vi "Big_LED_control.vi"() -> ()   [LabVIEW 2018]
uses:
  <instrlib>/niDCPower/nidcpower.llb/niDCPower Source Mode.ctl
  D:/#msp/LV/LED_CONTROL_big_LED_ophir_19.12_1/AT lib/AmateurStepperMotor.dll
  AT lib/AmateurStepperMotor.dll
  <instrlib>/niDMM/nidmm.llb/niDMM Function.ctl
  <instrlib>/niDMM/nidmm.llb/niDMM Resolution in Digits.ctl
  <instrlib>/niDCPower/nidcpower.llb/niDCPower Measurement Type.ctl
  <vilib>/Instr/_visa.llb/VISA Configure Serial Port (Instr).vi
  <instrlib>/niDMM/nidmm.llb/niDMM Configure Measurement Digits.vi
panel:
  in  "Tab Control 2":enum32{"Шаговик и офир", "Служебная область"}(tab)
  in  "milliseconds to wait":u32=1000
  in  "Go To":dbl
  out "Ophir 1 Char":dbl(graph)=7.0
  in  "DecelerationTime, s":dbl
  in  "AccelerationTime, s":dbl
  in  "HoldOn":bool
  in  "Ophir 1 units":string(combo)="1000" caption="Units"
  out "Ophir 1 Over Range":bool caption="Over Range"
  out "Ophir 1 Optical Power":dbl=7.0 caption="Power" format="%#_4g"
  out "Ophir 1 MAX":dbl=7.0200000000000005 caption="MAX" format="%#_5g"
  in  "Ophir 1 Clear":bool caption="Clear"
  in  "StepMultiplicationFactor":dbl=1.0
  in  "StepDivisor":i32(ring)=8 items=["D1"=1, "D2"=2, "D4"=4, "D8"=8, "D16"=16, "D32"=32]
  in  "Speed":dbl=1000.0
  in  "Погнали!":bool
  in  "Стоп GoTo":bool
  out "Готово":bool
  out "Position":dbl
  in  "Ophir 1 Info":u16(ring)=1 caption="Info" items=["Device : JUNO; s/n:903793", "Head : PD300R-3W   ; s/n:779628"]
  in  "new pos":dbl
  in  "set pos":bool
  out "Device Response":string="*\n"
  in  "Ophir 1 usb channel":i16 caption="usb channel"
  out "Ophir 1 dup Visa Session":refnum<visa-resource-name>="USB0::0x0BD3::0x0777::NI-VISA-60004::RAW" caption="dup Visa Session"
  in  "Ophir 1 Baud Rate (3:9600)":i16(ring)=3 caption="Baud Rate (3:9600)" items=["300", "1200", "4800", "9600", "19200", "38400"]
  out "Ophir 1 Real Optical Power":dbl=0.007 format="%.6e"
  in  "Ophir 1 GPIB Address (10)":string="10" caption="GPIB Address (10)"
  in  "Ophir 1 Port Number (default 2)":i16=1 caption="Port Number (default 2)" min=0 max=20
  in  "Ophir 1 Select Communication Protocol":u16(ring) caption="Select Communication Protocol" items=["USB", "RS232", "GPIB"]
  out "Ophir 1 error out":errorcluster caption="error out"
  in  "Ophir 1 error in (no error)":errorcluster caption="error in (no error)"
  in  "Ophir 1 Wait":u32=100 caption="Wait"
  out "IsOpen":bool=TRUE
  out "Ophir 1 Initialization":bool=TRUE caption="Initialization"
  in  "Tab Control":T1(tab)
  in  "POWER":bool
  in  "Стоп":bool
  in  "Resource Name":refnum<k15>="PXI1Slot2" caption="Источник питания"
  in  "Амперметр":refnum<k15>="PXI1Slot4" caption="NI DMM 1"
  in  "V_MB, V":dbl=5.0 caption="voltage level" format="%_6p"
  in  "curlim_V_MB, A":dbl=0.3 caption="current limit" format="%_6p"
  out "curmes_V_MB, A":dbl caption="measurement" format="%_6g"
  out "chart_0":dbl(graph)=-0.001986406197333734 caption="Waveform Chart 5"
  in  "voltlim_I_LED, V":dbl=2.0 caption="current limit" min=0.01 format="%_6p"
  in  "I_LED, A":dbl=0.005 caption="voltage level" format="%_6p"
  out "chart_1":dbl(graph) caption="Waveform Chart 5"
  out "voltmes_I_LED, V":dbl caption="measurement" format="%_6g"
  out "Current Char":dbl(graph)=0.0019995495676994324
  in  "Arduino":refnum<visa-resource-name>="COM14"
  in  "Сегменты":bool[](array[boolean])=[FALSE, FALSE, FALSE, FALSE, FALSE, FALSE, FALSE, FALSE, FALSE, FALSE, FALSE, FALSE, FALSE, FALSE, FALSE, FALSE, FALSE, FALSE]
  in  "Вольтметр":refnum<k15>="PXI1Slot5" caption="NI DMM 1"
  out "Voltage Char":dbl(graph)=nan
  in  "Port Name":string="COM7" caption="Порт шаговика"
  in  "wave_lenght":string="600"
  in  "Промер":bool caption="Промер сегмента"
  in  "NI DMM 1 Voltage Range 4":string(combo)="-1" caption="Range"
  in  "NI DMM 1 units 4":string(combo)="1" caption="Units"
  out "Voltage":dbl=nan format="%_6g"
  in  "NI DMM 1 Current Range 3":string(combo)="1" caption="Range"
  in  "NI DMM 1 units 3":string(combo)="1000" caption="Units"
  out "Current":dbl=0.0019995495676994324 format="%_6g"
  out "Разряд":dbl
  out "+/-":bool
  out "Power off":bool=TRUE
  in  "Command":string="Anode"
  in  "Записать":bool
  out "measure output file refnum":refnum<file>
  out "Voltage, V":dbl=nan caption="Measurement" format="%.5f"
  out "Current, A":dbl=1.9995495676994324e-06 caption="Measurement" format="%.5f"
  out "Тип индикатора":string="Anode"
  out "chart_2":dbl(graph)=4.286668577189643e-07
  in  "V_RES, V":dbl caption="voltage level" format="%_6p"
  out "curmes_V_RES, A":dbl caption="measurement" format="%_6g"
  in  "curlim_V_RES, A":dbl=0.1 caption="current limit" min=0.01 format="%_6p"
  in  "measure path":path=path "D:/NI LabVIEW/MultiOpto/MultiOpto_1.2/Logs/SEL"
  out "Enum":enum16{"Exit", "4", "Промер", "2", "1"}(ring)
  out "№ об-ца":dbl=-1.0
  out "Темп-ра":dbl=-1.0
  out "Сегмент":string
  # "Шаговик"
  # "Офир"
  # "Шаговик"
  # "Офир"
  # "position - это значение абсолютное"
  # "j"
  # "c"
  # "d"
  # "e"
  # "g"
  # "h"
  # "a"
  # "b"
  # "f"
  # "k"
  # "L"
  # "m"
  # "n"
  # "p"
  # "dp"
  # "all"
  # "V_MB 5 В\nогрничение 300 м\n\nV_LED 2,1 В\nограничение 200 м"
  # "единицы мА\nrange 1 А"
  # "1. каждый сегмент включаем по отдельности, резистором постраиваем ток до 10 мА\n2. напряжение V_LED при этом не меняется\n3. в такоом положении промеряем сегменты по отдельности\n4. для промера всего индикатора сразу подстраиваем напряжение при неизменном положении резисторов\n5. ток всех индикаторов = ток одного сегмента (10 мА) * число сегментов (15)\n6. добиваемся этого увеличением V_LED"
  # "единицы В\nrange AUTO"
  # "регклировка суммарного тока через индикатор"
  # "24.063\n\n     I          U\n20 мА  1.3 В\n20 мА  1.4 В\n 7 мА   1.15 В"
  # "24.064\n\n     I          U\n10 мА  2 В\n10 мА  2.15 В\n 7 мА   1.9 В"
  # "автоматизировать подбор напряжения по известному максимальному напряжению и току. ОС по току сегмента"
  # "Р1:  +25°C\nР2:  - 60°C\nР3:  +85°C"
  # "регулировать ток в зависимости от температуры.\nс ростом температуры растет ток.\nпид-регулятор??"
  # "0. ввести номер образца\n1. включить нужный сегмент\n2. ввести его в поле справа\n3. вести температуру в поле слева\n4. нажать кнопку \"промер сегмента\""
  # "\"опрашивать кнопки не чаще, чем раз в секунду. сейчас кликать можно чаще, они загорятся, но ничего не произойдет\""
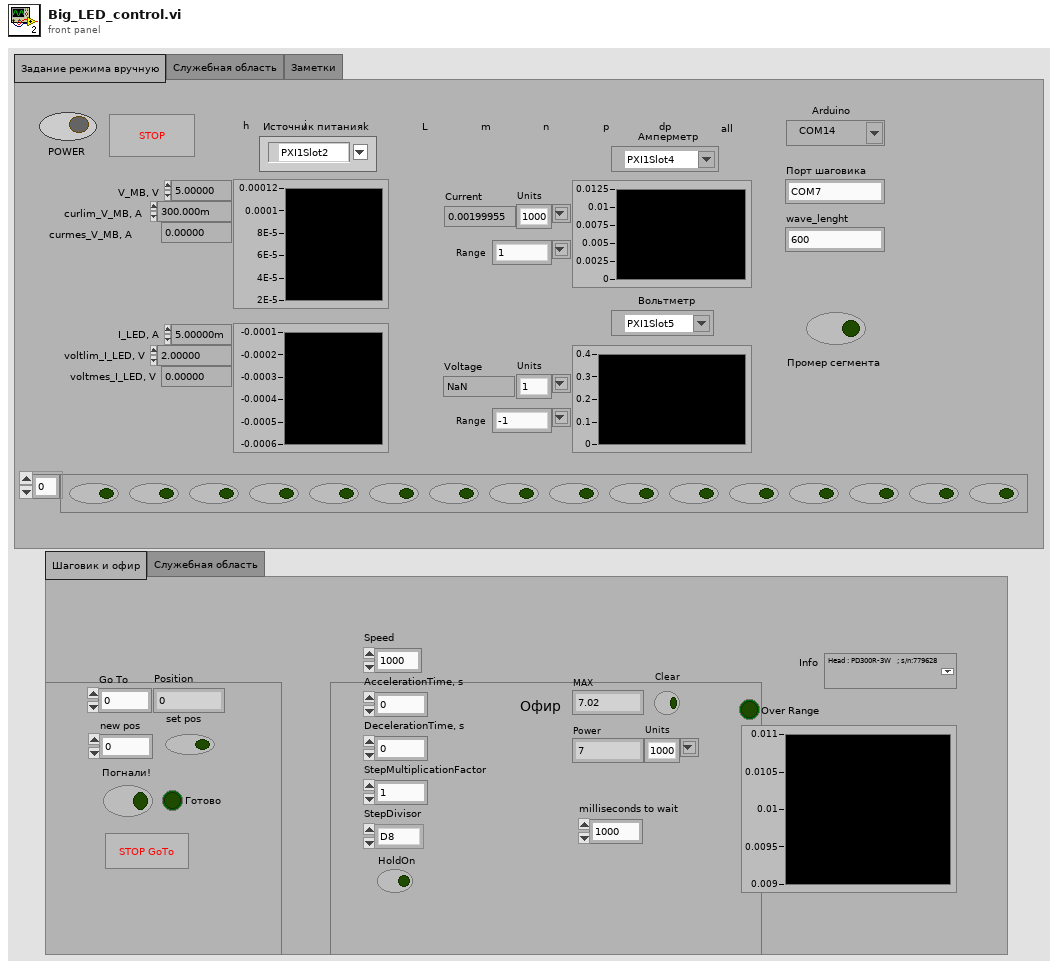
[diagram p1: front panel]
types:
  T1 = enum32{"Задание режима вручную", "Служебная область", "Заметки"}
  T2 = enum16{"open", "replace", "create", "open or create", "replace or create", "replace or create with confirmation"}
  T3 = typedef "niDCPower Source Mode.ctl" = i32
  T4 = typedef "niDCPower Measurement Type.ctl" = i32
  T5 = typedef "niDMM Function.ctl" = enum16{"DC Volts", "AC Volts", "DC Current", "AC Current", "2-wire Resistance", "4-wire Resistance", "Diode", "Frequency", "Period", "AC Volts DC Coupled", "Capacitance", "Inductance", "Temperature"}
  T6 = typedef "niDMM Resolution in Digits.ctl" = dbl
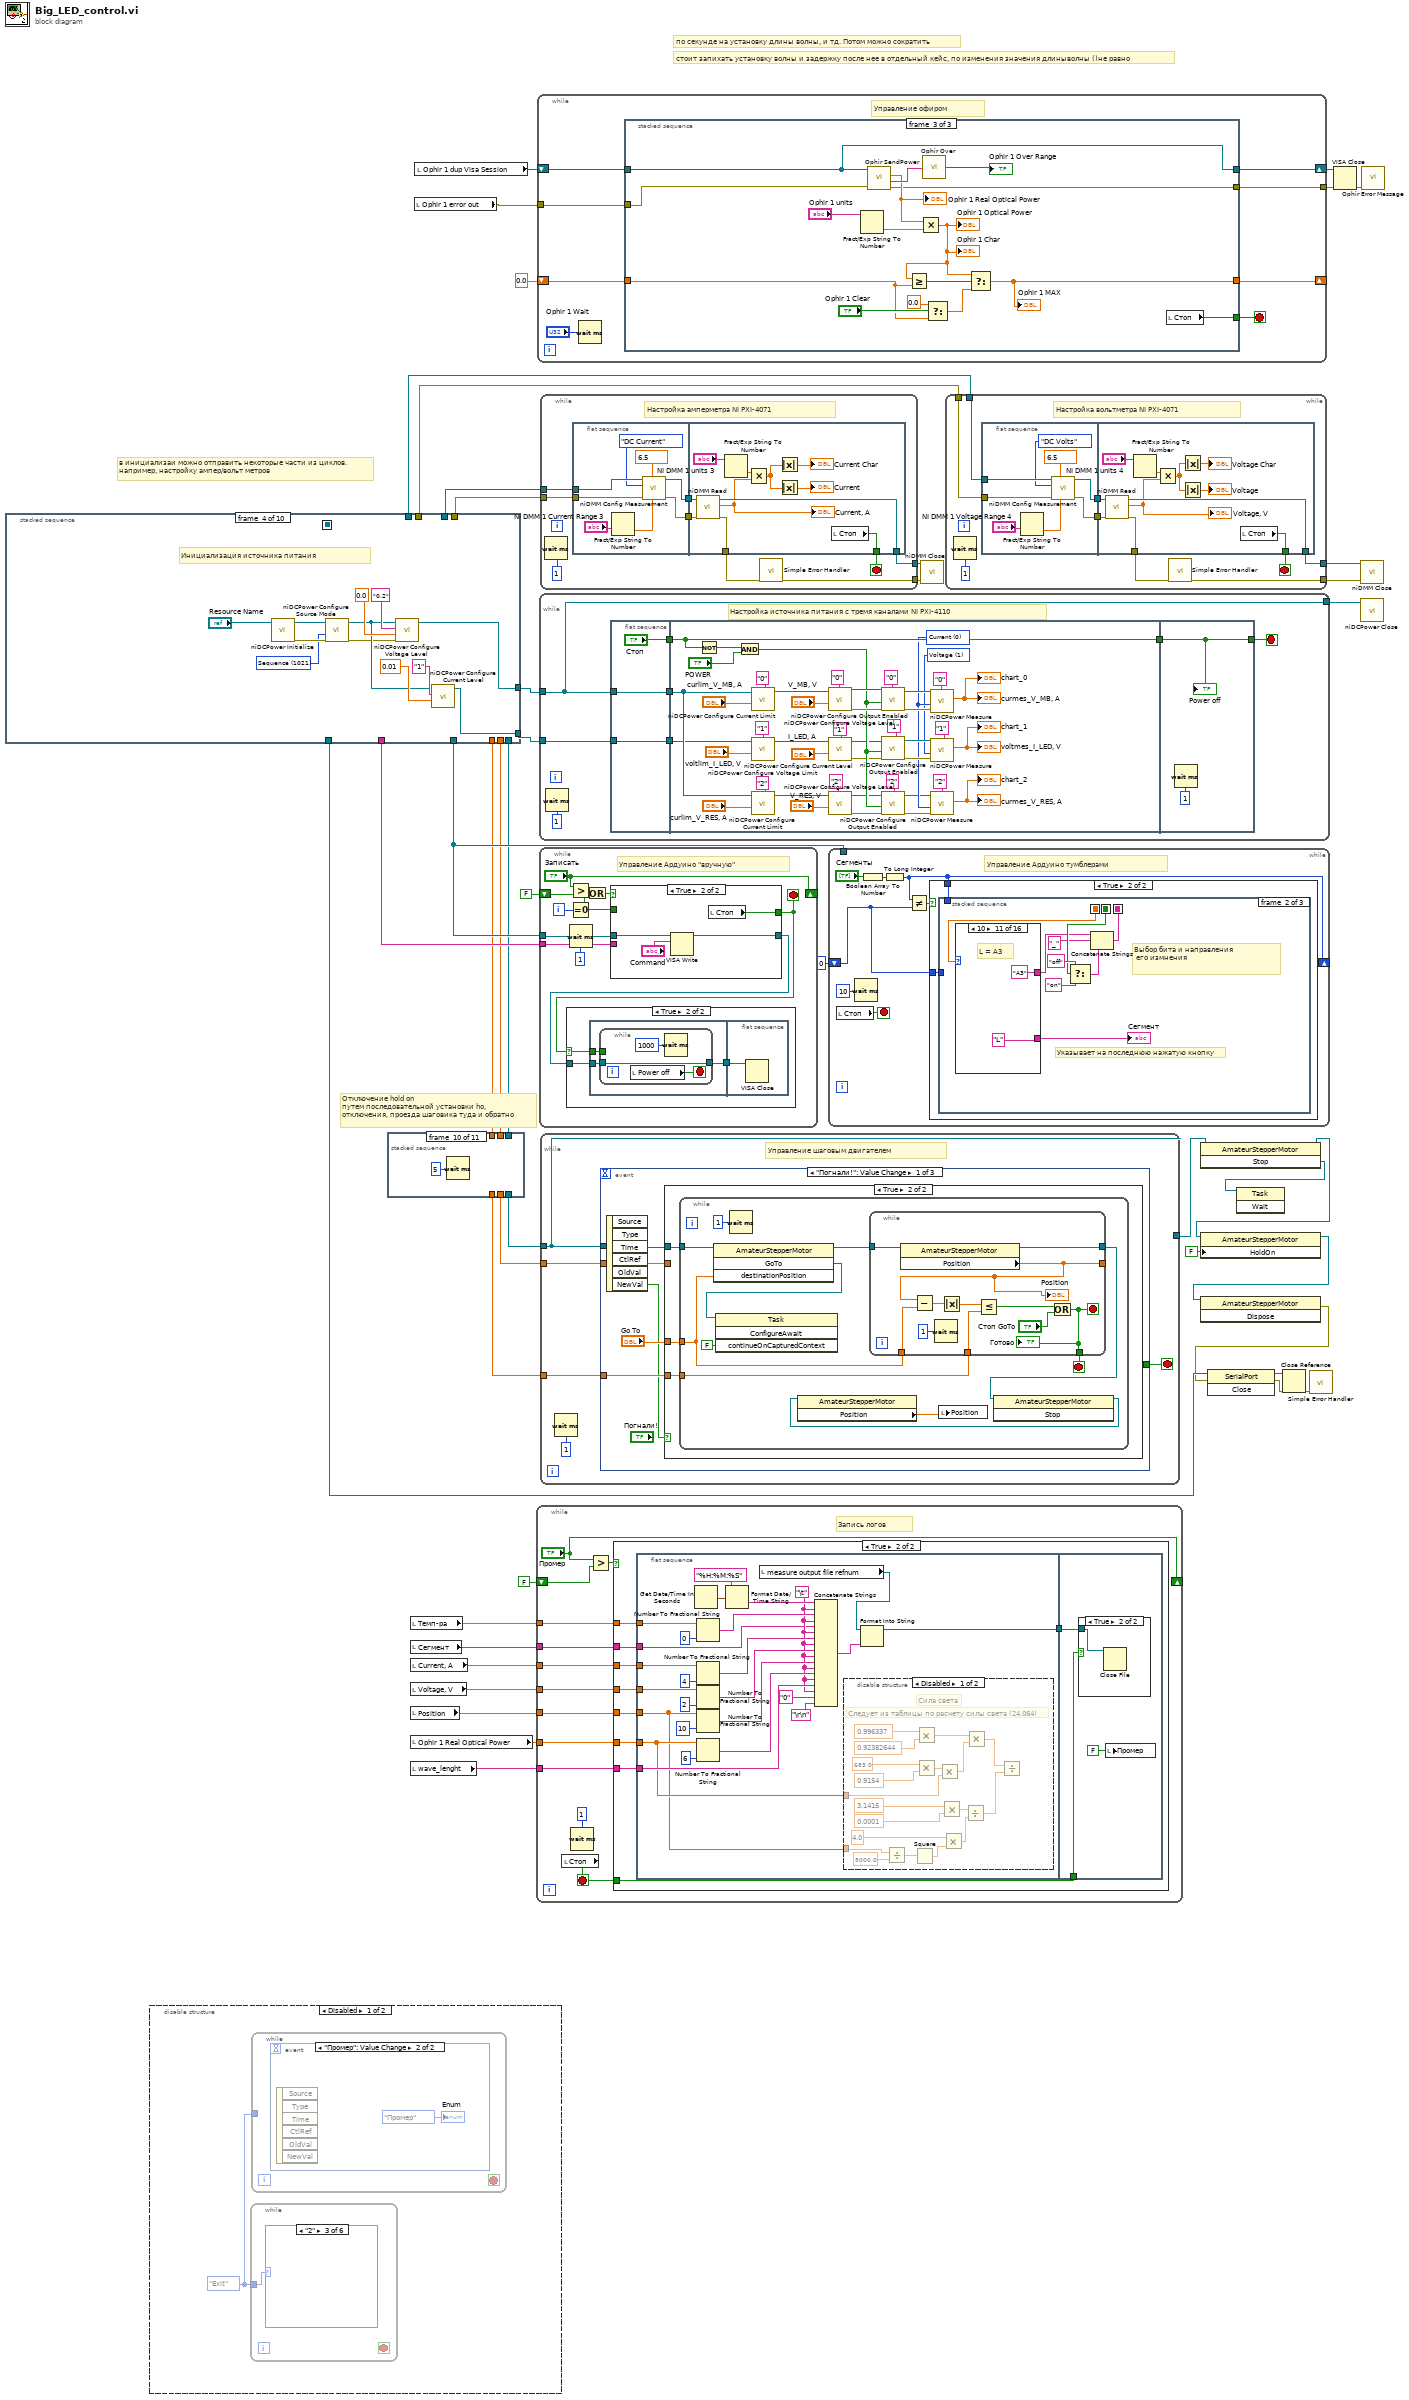
[diagram p0: block diagram]
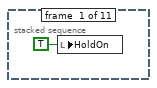
[diagram p2: hidden frame]
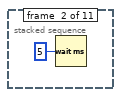
[diagram p3: hidden frame]
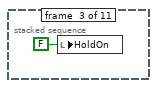
[diagram p4: hidden frame]
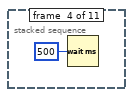
[diagram p5: hidden frame]
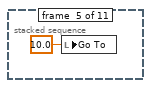
[diagram p6: hidden frame]
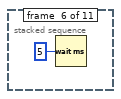
[diagram p7: hidden frame]
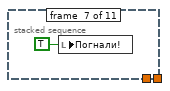
[diagram p8: hidden frame]
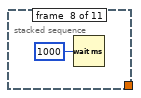
[diagram p9: hidden frame]
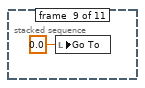
[diagram p10: hidden frame]
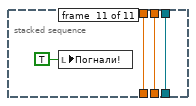
[diagram p11: hidden frame]
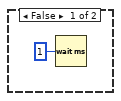
[diagram p12: hidden frame]
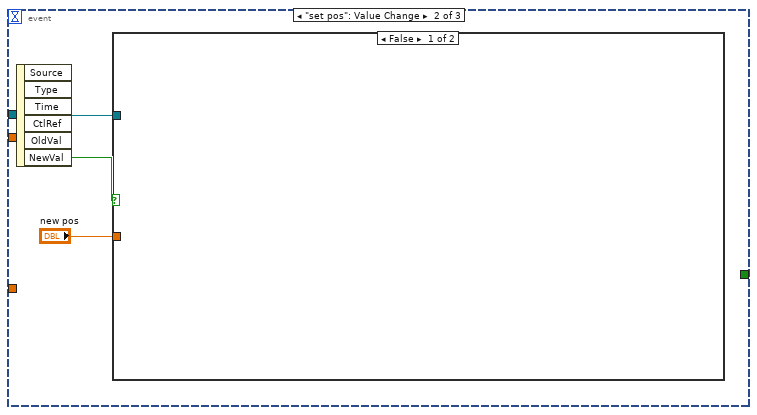
[diagram p13: hidden frame]
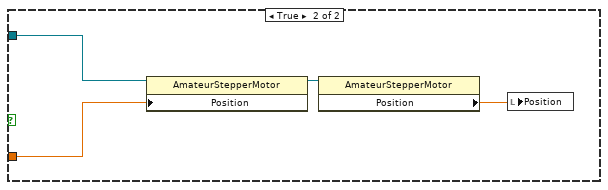
[diagram p14: hidden frame]
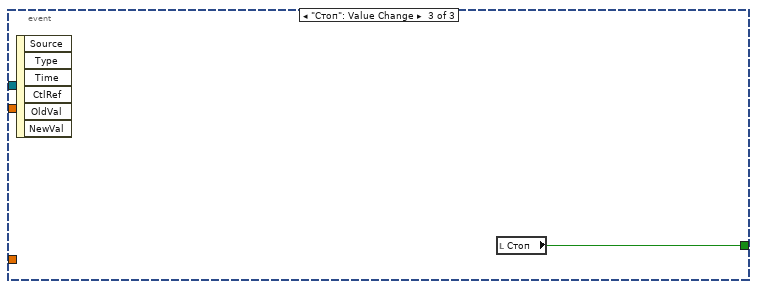
[diagram p15: hidden frame]
diagram:
  # "Отключение hold on\nпутем последовательной установки ho, \nотключения, проезда шаговика туда и обратно"
  # "в инициализаи можно отправить некоторые части из циклов.\nнапример, настройку ампер/вольт метров"
  # "стоит запихать установку волны и задержку после нее в отдельный кейс, по изменения значения длиныволны ()не равно"
  # "по секунде на установку длины волны, и тд. Потом можно сократить"
  n1 = stacked-sequence {
    seq-local: [_ _ _ _ _ _ w101 _ _ _] -> [_ _ _ _ _ _ _ w110 _ _]
    tunnel: [_ _ _ w67 _ _ _ _ _ _] -> w33
    tunnel: [_ w52 _ _ _ _ _ _ _ _] -> w45
    tunnel: [_ w51 _ _ _ _ _ _ _ _] -> w44
    tunnel: [_ _ _ _ w68 _ _ _ _ _] -> w41
    tunnel: [_ _ _ _ _ _ _ _ _ w150] -> w40
    tunnel: [_ _ w55 _ _ _ _ _ _ _] -> w39
    tunnel: [_ _ w54 _ _ _ _ _ _ _] -> w38
    tunnel: [_ _ _ _ _ _ _ w113 _ _] -> w1
    tunnel: [_ _ _ _ _ _ _ w111 _ _] -> w4
    tunnel: [_ _ _ _ _ _ _ w112 _ _] -> w6
    tunnel: [_ _ _ _ _ _ w91 _ _ _] -> w27
    tunnel: [_ _ _ w61 _ _ _ _ _ _] -> w10
    frame #0 {
      w46 = 0.0 ("currentmes_2")
      w47 = FALSE ("Стоп")
      # "Обнуление переменных"
      n2 = local write "POWER"(w47) -> ()
      n3 = local write "Стоп"(w47) -> ()
      n4 = local write "+/-"(w47) -> ()
      n5 = local write "Погнали!"(w47) -> ()
      n6 = local write "Готово"(w47) -> ()
      n7 = local write "Стоп GoTo"(w47) -> ()
      n8 = local write "Go To"(w46) -> ()
      n9 = local write "curmes_V_MB, A"(w46) -> ()
      n10 = local write "curmes_V_RES, A"(w46) -> ()
      n11 = local write "Current"(w46) -> ()
      n12 = local write "Разряд"(w46) -> ()
      n13 = local write "voltmes_I_LED, V"(w46) -> ()
      n14 = local write "Сегменты"(bool[] [FALSE, FALSE, FALSE, FALSE, FALSE, FALSE, FALSE, FALSE, FALSE, FALSE, FALSE, FALSE, FALSE, FALSE, FALSE, FALSE, FALSE, FALSE] ("Сегменты")) -> ()
      n15 = local write "Command"("zero" ("Command 2")) -> ()
    }
    frame #1 {
      # "Инициализация амперметра"
      n16 = call <instrlib>:"niDMM Initialize.vi"("Instrument Descriptor"="Амперметр") -> ("error out"=w52:errorcluster, "instrument handle out"=w51:refnum<k15>)  [unwired: 9 in]
    }
    frame #2 {
      # "Инициализация вольтметра"
      n17 = call <instrlib>:"niDMM Initialize.vi"("Instrument Descriptor"="Вольтметр") -> ("error out"=w54:errorcluster, "instrument handle out"=w55:refnum<k15>)  [unwired: 9 in]
    }
    frame #3 {
      w56 = T3 1021 items=["Single Point"=1020, "Sequence"=1021] ("source mode")
      # "Инициализация источника питания"
      n18 = call <instrlib>:"niDCPower Initialize.vi"("resource name"="Resource Name") -> ("error out"=w59:errorcluster, "instrument handle out"=w60:refnum<k15>)  [unwired: 3 in, 6 out]
      n19 = call <instrlib>:"niDCPower Configure Source Mode.vi"("error in (no error)"=w59, "source mode"=w56, "instrument handle"=w60) -> ("error out"=w57:errorcluster, "instrument handle out"=w58:refnum<k15>)  [unwired: 7 out]
      n20 = call <instrlib>:"niDCPower Configure Voltage Level.vi"("error in (no error)"=w57, "voltage level"=0.0, "channel name"="0,2", "instrument handle"=w58) -> ("instrument handle out"=w67:refnum<k15>)  [unwired: 6 in, 1 out]
      n21 = call <instrlib>:"niDCPower Configure Current Level.vi"("current level"=0.01, "channel name"="1", "instrument handle"=w58) -> ("instrument handle out"=w61:refnum<k15>)  [unwired: 7 in, 1 out]
    }
    frame #4 {
      # "Инициализация Ардуино"
      n22 = call-poly "VISA Configure Serial Port"("VISA resource name"="Arduino", "baud rate (9600)"=u32 9600) -> ("VISA resource name out"=w68:refnum<visa-resource-name>)  [unwired: 12 in, 1 out]
    }
    frame #5 {
      # "Инициализация офира"
      n23 = call "Ophir InitCom.vi"("GPIB Address (default 10)"="Ophir 1 GPIB Address (10)", "Communication (default USB 0)"="Ophir 1 Select Communication Protocol", "USB Channel number (default 0)"="Ophir 1 usb channel", "Port Number (default 2)"="Ophir 1 Port Number (default 2)", "error in (no error)"="Ophir 1 error in (no error)", "Baud Rate (3:9600)"="Ophir 1 Baud Rate (3:9600)") -> ("dup Visa Session"=w77:refnum<visa-resource-name>, "error out"=w76:errorcluster)  [unwired: 1 out]
      n24 = call "Ophir InstrInfo.vi"("Visa Session"=w77, "error in (no error)"=w76) -> ("dup Visa Session"=w89:refnum<visa-resource-name>, "Instrument Info"=w71:string, "error out"=w87:errorcluster)
      n25 = call "Ophir HeadInfo.vi"("Visa Session"=w89, "error in (no error)"=w87) -> ("error out"=w86:errorcluster, "dup Visa Session"=w88:refnum<visa-resource-name>, "Head Info"=w85:string)  [unwired: 6 out]
      n26 = call "Ophir InfoStrings.vi"("error in (no error)"=w86, "Head Info"=w85, "Instrument Info"=w71) -> ("error out"=w84:errorcluster, "Strings Array"=w83:string[])
      n27 = property on="Ophir 1 Info" class="Ring (strict)"("Strings []"=w83) -> ()  [unwired: 2 in, 2 out]
      n28 = call "Ophir ConfigDevice.vi"("Visa Session"=w88, "Measure Choice (0:Power)"=u16 0, "error in (no error)"=w84) -> ("dup Visa Session"=→"Ophir 1 dup Visa Session":refnum<visa-resource-name>, "OK ?"=→"Ophir 1 Initialization":bool, "error out"=→"Ophir 1 error out":errorcluster)  [unwired: 1 out]
    }
    frame #6 {
      w95 = 100 ("WriteTimeout")
      w100 = 1 items=["None", "One", "Two", "OnePointFive"] ("stopBits")
      w97 = 0 items=["None", "Odd", "Even", "Mark", "Space"] ("parity")
      # "убрали открытие порта. шаговик его и так сам откроет"
      # "Инициализация шаговика ч.1"
      n29 = constructor class="SerialPort"("portName"="Port Name", "baudRate"=57600, "parity"=w97, "dataBits"=8, "stopBits"=w100) -> (reference out=w94:refnum<k24>, error out=w93:errorcluster)  [unwired: 3 in, 6 out]
      n30 = property class="SerialPort"(reference=w94, error in=w93, "WriteTimeout"=w95, "ReadTimeout"=w95) -> (reference out=w91:refnum<k24>)  [unwired: 1 out]
      n31 = constructor class="AmateurStepperMotor"("serialPort"=w91) -> (reference out=w101:refnum<k24>, error out=w92:errorcluster)  [unwired: 3 in, 2 out]
      n32 = flat-sequence {
        tunnel: w92 -> [_]
        tunnel: w91 -> [w103]
        frame #0 {
          n33 = property class="SerialPort"(reference=w103) -> ("IsOpen"=→"IsOpen":bool)  [unwired: 1 in, 2 out]
        }
      }
    }
    frame #7 {
      # "стоит допустить изменение\nтих параметров в цикле, а не только \nпри инициализации"
      # "это те самые 50 шагов за мм"
      # "Инициализация шаговика ч.2"
      n34 = property class="AmateurStepperMotor"(reference=w110, "Speed"="Speed", "StepDivisor"="StepDivisor", "StepMultiplicationFactor"="StepMultiplicationFactor", "AccelerationTime"="AccelerationTime, s", "DecelerationTime"="DecelerationTime, s", "HoldOn"="HoldOn") -> (reference out=w113:refnum<k24>, "Position"=w111:dbl, "PositioningPrecision"=w112:dbl)  [unwired: 1 in, 1 out]
    }
    frame #8 {
      w119 = "\t"
      # "Инициализация логов"
      n35 = local read "№ об-ца"() -> (w115:dbl)
      n36 = Number To Fractional String(number=w115, precision (6)=i16 0) -> (F-format string=w116:string)  [unwired: 2 in]
      n37 = Get Date/Time In Seconds() -> (seconds since 1Jan1904=w137:timestamp)
      n38 = Build Path(base path="measure path", name or relative path=w116) -> (appended path=w133:path)
      n39 = call <vilib>:"Check if File or Folder Exists.vi"("path"=w133) -> ("file or folder exists?"=w134:bool, "dup path"=w135:path)  [unwired: 8 in, 1 out]
      n40 = Format Date/Time String(time format string (%c)="MES %d %m %y %H.%M.%S", seconds (now)=w137) -> (date/time string=w138:string)  [unwired: 1 in]
      n41 = case shown="False" w134 {
        tunnel: w135 -> [w146 w147]
        tunnel: [w145 w147] -> w136
        frame False {
          n42 = Create Folder(path (use dialog)=w146) -> (created path=w145:path)  [unwired: 2 in, 2 out]
        }
        frame True {
        }
      }
      n43 = Concatenate Strings(w138, ".xls" ("string")) -> (w139:string)
      n44 = Build Path(base path=w136, name or relative path=w139) -> (appended path=w140:path)
      n45 = Open/Create/Replace File(file path (use dialog)=w140, operation (0:open)=T2."open or create", access (0:read/write)=enum16{"read/write", "read-only", "write-only"}."read/write") -> (refnum out=w141:refnum<file>)  [unwired: 3 in, 2 out]
      n46 = Set File Position(refnum=w141, from (0:start)=enum16{"start", "end", "current"}."end") -> (refnum out=w143:refnum<file>)  [unwired: 2 in, 1 out]
      n47 = Format Into String(initial string=w143, "Time" ("string"), w119, "Temperature, C" ("string"), w119, "Segment" ("string"), w119, "Current, mA" ("string"), w119, "Voltage, V" ("input 7"), w119, "Distance, m" ("string"), w119, "Power, W " ("string"), w119, "Wavelenght, nm" ("input 17"), w119, "Candlepower, kd" ("string"), "\r\n") -> (resulting string=→"measure output file refnum":refnum<file>)  [unwired: 2 in, 1 out]
    }
    frame #9 {
      # "Begin VI: ОК или ОА?"
      n48 = call "Begin.vi"() -> ("Темп-ра"=→"Темп-ра":dbl, "№ об-ца"=→"№ об-ца":dbl, "String"=w150:string)  [unwired: 6 in]
      "Тип индикатора" <- w150
      n49 = local write "Command"(w150) -> ()
    }
  }
  n50 = disable-structure shown="Disabled" {
    frame Disabled {
      w151 = enum16{"Exit", "4", "Промер", "2", "1"}."Exit"
      n51 = while {
        tunnel: w151 -> [w152]
        stop <- _ stop-if-true
        n52 = case shown="\"2\"" w152 {
          frame "Exit", Default {
          }
          frame "4" {
          }
          frame "2" {
          }
          frame "2" {
          }
          frame "1" {
          }
          frame "Промер" {
          }
        }
      }
      n53 = while {
        tunnel: w151 -> [_]
        stop <- _ stop-if-true
        n54 = event shown="[1] \"Промер\": Value Change" {
          selector: _ -> [_ _]
          dyn-events: _ -> [_ _]
          timeout: _ -> [_ _]
          event Timeout {
            n55 = event-data() -> ()  [unwired: 1 in, 3 out]
          }
          event "Промер": Value Change {
            n56 = event-data() -> ()  [unwired: 1 in, 6 out]
            "Enum" <- enum16{"Exit", "4", "Промер", "2", "1"}."Промер" ("Enum")
          }
        }
      }
    }
    frame Enabled {
    }
  }
  n57 = stacked-sequence {
    tunnel: w6 -> [_ _ _ _ _ _ _ _ _ _ w166]
    tunnel: [_ _ _ _ _ _ _ _ _ _ w166] -> w5
    tunnel: w4 -> [_ _ _ _ _ _ _ _ _ _ w165]
    tunnel: [_ _ _ _ _ _ _ _ _ _ w165] -> w3
    tunnel: [_ _ _ _ _ _ _ _ _ _ w164] -> w2
    tunnel: w1 -> [_ _ _ _ _ _ _ _ _ _ w164]
    frame #0 {
      n58 = local write "HoldOn"(TRUE ("HoldOn")) -> ()
    }
    frame #1 {
      n59 = Wait (ms)(milliseconds to wait=u32 5) -> ()  [unwired: 1 out]
    }
    frame #2 {
      n60 = local write "HoldOn"(FALSE ("HoldOn")) -> ()
    }
    frame #3 {
      n61 = Wait (ms)(milliseconds to wait=u32 500) -> ()  [unwired: 1 out]
    }
    frame #4 {
      n62 = local write "Go To"(10.0 ("Go To")) -> ()
    }
    frame #5 {
      n63 = Wait (ms)(milliseconds to wait=u32 5) -> ()  [unwired: 1 out]
    }
    frame #6 {
      n64 = local write "Погнали!"(TRUE ("Погнали!")) -> ()
    }
    frame #7 {
      n65 = Wait (ms)(milliseconds to wait=u32 1000) -> ()  [unwired: 1 out]
    }
    frame #8 {
      n66 = local write "Go To"(0.0 ("Go To")) -> ()
    }
    frame #9 {
      n67 = Wait (ms)(milliseconds to wait=u32 5) -> ()  [unwired: 1 out]
    }
    frame #10 {
      n68 = local write "Погнали!"(TRUE ("Погнали!")) -> ()
    }
  }
  n69 = local read "Темп-ра"() -> (w8:dbl)
  n70 = local read "Сегмент"() -> (w7:string)
  n71 = local read "Current, A"() -> (w26:dbl)
  n72 = local read "Voltage, V"() -> (w25:dbl)
  n73 = local read "Position"() -> (w24:dbl)
  n74 = local read "Ophir 1 Real Optical Power"() -> (w23:dbl)
  n75 = local read "wave_lenght"() -> (w22:string)
  n76 = local read "Ophir 1 error out"() -> (w31:errorcluster)
  n77 = local read "Ophir 1 dup Visa Session"() -> (w32:refnum<visa-resource-name>)
  n78 = while {
    tunnel: w26 -> [w179]
    tunnel: w25 -> [w178]
    tunnel: w24 -> [w177]
    tunnel: w23 -> [w176]
    tunnel: w22 -> [w175]
    shift-right: ["Промер"] -> _
    shift-left: FALSE ("Промер сегмента") -> [w172]
    tunnel: w8 -> [w169]
    tunnel: w7 -> [w168]
    stop <- w170 stop-if-true
    # "Запиcь логов"
    n79 = local read "Стоп"() -> (w170:bool)
    n80 = Wait (ms)(milliseconds to wait=u32 1) -> ()  [unwired: 1 out]
    n81 = Greater?(x="Промер", y=w172) -> (0:w173:bool)
    n82 = case shown="True" w173 {
      tunnel: w179 -> [_ w188]
      tunnel: w178 -> [_ w187]
      tunnel: w177 -> [_ w184]
      tunnel: w176 -> [_ w185]
      tunnel: w175 -> [_ w186]
      tunnel: w170 -> [_ w182]
      tunnel: w169 -> [_ w181]
      tunnel: w168 -> [_ w180]
      frame False {
      }
      frame True {
        n83 = flat-sequence {
          tunnel: w188 -> [w206]
          tunnel: w187 -> [w205]
          tunnel: w186 -> [w203]
          tunnel: w185 -> [w202]
          tunnel: w184 -> [w201]
          tunnel: [w196] -> w183
          tunnel: w181 -> [w195]
          tunnel: w180 -> [w189]
          tunnel: w183 -> [w236]
          tunnel: w182 -> [w235]
          frame #0 {
            w191 = "\t"
            n84 = Get Date/Time In Seconds() -> (seconds since 1Jan1904=w214:timestamp)
            n85 = Number To Fractional String(number=w195, precision (6)=i16 0) -> (F-format string=w193:string)  [unwired: 2 in]
            n86 = Number To Fractional String(number=w206, precision (6)=i16 4) -> (F-format string=w209:string)  [unwired: 2 in]
            n87 = Number To Fractional String(number=w205, precision (6)=i16 2) -> (F-format string=w208:string)  [unwired: 2 in]
            n88 = Number To Fractional String(number=w201, precision (6)=i16 10) -> (F-format string=w207:string)  [unwired: 2 in]
            n89 = Number To Fractional String(number=w202, precision (6)=i16 6) -> (F-format string=w204:string)  [unwired: 2 in]
            n90 = Format Date/Time String(time format string (%c)="%H:%M:%S", seconds (now)=w214) -> (date/time string=w212:string)  [unwired: 1 in]
            n91 = local read "measure output file refnum"() -> (w210:refnum<file>)
            n92 = Concatenate Strings(w212, w191, w193, w191, w189, w191, w209, w191, w208, w191, w207, w191, w204, w191, w203, w191, "0" ("string"), "\r\n") -> (w211:string)
            n93 = disable-structure shown="Disabled" {
              disable-tunnel: w202 -> [w226 _]
              disable-tunnel: w201 -> [w216 _]
              frame Disabled {
                # "Сила света"
                # "Следует из таблицы по расчету силы света (24.064)"
                n94 = Divide(x=w216, y=5000.0) -> (x/y=w218:dbl)
                n95 = Square(x=w218) -> (x^2=w217:dbl)
                n96 = Multiply(x=0.996337, y=0.92382644) -> (x*y=w231:dbl)
                n97 = Multiply(x=683.0, y=0.9154) -> (x*y=w227:dbl)
                n98 = Multiply(x=w227, y=w226) -> (x*y=w225:dbl)
                n99 = Multiply(x=3.1415, y=0.0001) -> (x*y=w221:dbl)
                n100 = Multiply(x=4.0, y=w217) -> (x*y=w220:dbl)
                n101 = Divide(x=w221, y=w220) -> (x/y=w222:dbl)
                n102 = Multiply(x=w231, y=w225) -> (x*y=w230:dbl)
                n103 = Divide(x=w230, y=w222) -> ()  [unwired: 1 out]
              }
              frame Enabled {
              }
            }
            n104 = Format Into String(initial string=w210, w211) -> (resulting string=w196:refnum<file>)  [unwired: 2 in, 1 out]
          }
          frame #1 {
            n105 = case shown="True" w235 {
              tunnel: w236 -> [_ w237]
              frame False {
              }
              frame True {
                n106 = Close File(refnum=w237) -> ()  [unwired: 1 in, 2 out]
              }
            }
            n107 = local write "Промер"(FALSE ("Промер")) -> ()
          }
        }
      }
    }
  }
  n108 = while {
    tunnel: w31 -> [w244]
    shift-right: [w240] -> _
    shift-left: 0.0 ("t") -> [w243]
    shift-right: [w241] -> w20
    shift-left: w32 -> [w245]
    tunnel: [w239] -> w19
    stop <- w238 stop-if-true
    # "Управление офиром"
    n109 = Wait (ms)(milliseconds to wait="Ophir 1 Wait") -> ()  [unwired: 1 out]
    n110 = stacked-sequence {
      tunnel: w245 -> [w249 _ w252]
      tunnel: w244 -> [w248 _ w254]
      tunnel: w243 -> [_ _ w255]
      tunnel: [_ _ w252] -> w241
      tunnel: [_ _ w256] -> w240
      tunnel: [_ _ w253] -> w239
      tunnel: [_ _ w251] -> w238
      frame #0 {
        n111 = call "light_setWaveLenght.vi"("error in (no error)"=w248, "Visa Session"=w249, "wave_lenght"="wave_lenght") -> ("Device Response"=→"Device Response":string)  [unwired: 6 in, 2 out]
      }
      frame #1 {
        n112 = Wait (ms)(milliseconds to wait="milliseconds to wait") -> ()  [unwired: 1 out]
      }
      frame #2 {
        n113 = Fract/Exp String To Number(string="Ophir 1 units") -> (number=w259:dbl)  [unwired: 3 in, 1 out]
        n114 = call "Ophir SendPower.vi"("Visa Session"=w252, "error in (no error)"=w254) -> ("Value Number"=w258:dbl, "Value String"=w265:string, "error out"=w253:errorcluster)  [unwired: 1 out]
        "Ophir 1 Real Optical Power" <- w258
        n115 = Multiply(x=w258, y=w259) -> (x*y=w262:dbl)
        "Ophir 1 Char" <- w262
        "Ophir 1 Optical Power" <- w262
        n116 = Greater Or Equal?(x=w262, y=w255) -> (x >= y?=w263:bool)
        n117 = call "Ophir Over.vi"("Value String"=w265) -> ("Overrange"=→"Ophir 1 Over Range":bool)
        n118 = Select(t=0.0, s="Ophir 1 Clear", f=w255) -> (s? t:f=w261:dbl)
        n119 = Select(t=w262, s=w263, f=w261) -> (s? t:f=w256:dbl)
        "Ophir 1 MAX" <- w256
        n120 = local read "Стоп"() -> (w251:bool)
      }
    }
  }
  n121 = while {
    tunnel: w33 -> [w271]
    tunnel: [w271] -> w42
    tunnel: w10 -> [w268]
    stop <- w267 stop-if-true
    # "Настройка источника питания с тремя каналами NI PXI-4110"
    n122 = Wait (ms)(milliseconds to wait=u32 1) -> ()  [unwired: 1 out]
    n123 = flat-sequence {
      tunnel: w271 -> [w277]
      tunnel: [w277] -> w273
      tunnel: ["Стоп"] -> w272
      tunnel: [w275] -> w269
      tunnel: w268 -> [w275]
      tunnel: w273 -> [w311]
      tunnel: w272 -> [w321]
      tunnel: [w321] -> w270
      tunnel: w269 -> [w305]
      tunnel: [w323] -> w267
      tunnel: w270 -> [w323]
      frame #0 {
      }
      frame #1 {
        w298 = T4 1 items=["Current", "Voltage"] ("measurement type")
        w310 = T4 0 items=["Current", "Voltage"] ("measurement type")
        n124 = Not(x=w321) -> (.not. x?=w320:bool)
        n125 = And(x=w320, y="POWER") -> (x .and. y?=w308:bool)
        n126 = call <instrlib>:"niDCPower Configure Current Limit.vi"("current limit"="curlim_V_MB, A", "channel name"="0", "instrument handle"=w311) -> ("instrument handle out"=w296:refnum<k15>)  [unwired: 7 in, 1 out]
        n127 = call <instrlib>:"niDCPower Configure Voltage Limit.vi"("voltage limit"="voltlim_I_LED, V", "channel name"="1", "instrument handle"=w305) -> ("instrument handle out"=w302:refnum<k15>)  [unwired: 7 in, 1 out]
        n128 = call <instrlib>:"niDCPower Configure Current Limit.vi"("current limit"="curlim_V_RES, A", "channel name"="2", "instrument handle"=w311) -> ("instrument handle out"=w287:refnum<k15>)  [unwired: 7 in, 1 out]
        n129 = call <instrlib>:"niDCPower Configure Voltage Level.vi"("voltage level"="V_MB, V", "channel name"="0", "instrument handle"=w296) -> ("error out"=w316:errorcluster, "instrument handle out"=w315:refnum<k15>)  [unwired: 7 in]
        n130 = call <instrlib>:"niDCPower Configure Current Level.vi"("current level"="I_LED, A", "channel name"="1", "instrument handle"=w302) -> ("error out"=w300:errorcluster, "instrument handle out"=w303:refnum<k15>)  [unwired: 7 in]
        n131 = call <instrlib>:"niDCPower Configure Voltage Level.vi"("voltage level"="V_RES, V", "channel name"="2", "instrument handle"=w287) -> ("error out"=w289:errorcluster, "instrument handle out"=w288:refnum<k15>)  [unwired: 7 in]
        n132 = call <instrlib>:"niDCPower Configure Output Enabled.vi"("error in (no error)"=w316, "output enabled"=w308, "channel name"="0", "instrument handle"=w315) -> ("error out"=w313:errorcluster, "instrument handle out"=w314:refnum<k15>)  [unwired: 6 in]
        n133 = call <instrlib>:"niDCPower Configure Output Enabled.vi"("error in (no error)"=w300, "output enabled"=w308, "channel name"="1", "instrument handle"=w303) -> ("error out"=w318:errorcluster, "instrument handle out"=w317:refnum<k15>)  [unwired: 6 in]
        n134 = call <instrlib>:"niDCPower Configure Output Enabled.vi"("error in (no error)"=w289, "output enabled"=w308, "channel name"="2", "instrument handle"=w288) -> ("error out"=w285:errorcluster, "instrument handle out"=w284:refnum<k15>)  [unwired: 6 in]
        n135 = call <instrlib>:"niDCPower Measure.vi"("error in (no error)"=w313, "measurement type"=w310, "channel name"="0", "instrument handle"=w314) -> ("measurement"=→"curmes_V_MB, A" →"chart_0":dbl)  [unwired: 5 in, 2 out]
        n136 = call <instrlib>:"niDCPower Measure.vi"("error in (no error)"=w318, "measurement type"=w298, "channel name"="1", "instrument handle"=w317) -> ("measurement"=→"chart_1" →"voltmes_I_LED, V":dbl)  [unwired: 5 in, 2 out]
        n137 = call <instrlib>:"niDCPower Measure.vi"("error in (no error)"=w285, "measurement type"=w310, "channel name"="2", "instrument handle"=w284) -> ("measurement"=→"curmes_V_RES, A" →"chart_2":dbl)  [unwired: 5 in, 2 out]
      }
      frame #2 {
        n138 = Wait (ms)(milliseconds to wait=u32 1) -> ()  [unwired: 1 out]
        "Power off" <- w323
      }
    }
  }
  n139 = while {
    tunnel: w41 -> [w331]
    shift-right: ["Записать"] -> _
    shift-left: FALSE ("Записать") -> [w333]
    tunnel: w40 -> [w329]
    i -> [w330]
    stop <- w324 stop-if-true
    # "Управление Ардуино \"вручную\""
    n140 = Greater?(x="Записать", y=w333) -> (0:w327:bool)
    n141 = Equal To 0?(x=w330) -> (x = 0?=w326:bool)
    n142 = Wait (ms)(milliseconds to wait=u32 1) -> ()  [unwired: 1 out]
    n143 = Or(x=w327, y=w326) -> (x .or. y?=w328:bool)
    n144 = case shown="True" w328 {
      tunnel: w331 -> [w345 w350]
      tunnel: [w346 w349] -> w324
      tunnel: w329 -> [_ _]
      tunnel: w326 -> [_ _]
      tunnel: [w345 w347] -> w325
      frame False {
        n145 = local read "Стоп"() -> (w346:bool)
      }
      frame True {
        n146 = VISA Write(VISA resource name=w350, write buffer="Command") -> (VISA resource name out=w347:refnum<visa-resource-name>)  [unwired: 1 in, 2 out]
        n147 = local read "Стоп"() -> (w349:bool)
      }
    }
    n148 = case shown="True" w324 {
      selector: w324 -> [_ w335]
      tunnel: w325 -> [_ w337]
      frame False {
      }
      frame True {
        n149 = flat-sequence {
          tunnel: w337 -> [w340]
          tunnel: [w339] -> w336
          tunnel: w335 -> [w338]
          tunnel: w336 -> [w344]
          frame #0 {
            n150 = while {
              tunnel: w340 -> [w343]
              tunnel: [w343] -> w339
              tunnel: w338 -> [_]
              stop <- w341 stop-if-true
              n151 = local read "Power off"() -> (w341:bool)
              n152 = Wait (ms)(milliseconds to wait=u32 1000) -> ()  [unwired: 1 out]
            }
          }
          frame #1 {
            n153 = VISA Close(VISA resource name=w344) -> ()  [unwired: 1 in, 1 out]
          }
        }
      }
    }
  }
  n154 = while {
    tunnel: [w357] -> w34
    tunnel: w44 -> [w355]
    tunnel: w45 -> [w354]
    tunnel: [w351] -> w35
    stop <- w353 stop-if-true
    # "Настройка амперметра NI PXI-4071"
    n155 = Wait (ms)(milliseconds to wait=u32 1) -> ()  [unwired: 1 out]
    n156 = flat-sequence {
      tunnel: [w364] -> w359
      tunnel: w355 -> [w362]
      tunnel: w354 -> [w366]
      tunnel: [w363] -> w358
      tunnel: w359 -> [w375]
      tunnel: w358 -> [w378]
      tunnel: [w374] -> w353
      tunnel: [w373] -> w351
      tunnel: [w372] -> w352
      frame #0 {
        w360 = T6 6.5 items=["3 1/2"=3.5, "4 1/2"=4.5, "5 1/2"=5.5, "6 1/2"=6.5, "7 1/2"=7.5] ("Resolution in Digits")
        n157 = Fract/Exp String To Number(string="NI DMM 1 Current Range 3") -> (number=w365:dbl)  [unwired: 3 in, 1 out]
        n158 = call-poly <instrlib>:"niDMM Config Measurement.vi"("Range"=w365, "Resolution in Digits"=w360, "error in (no error)"=w366, "Function"=niDMM_Function."DC Current" ("Measurement Type"), "instrument handle"=w362) -> ("error out"=w363:errorcluster, "instrument handle out"=w364:refnum<k15>)  [unwired: 5 in]
      }
      frame #1 {
        n159 = call <instrlib>:"niDMM Read.vi"("error in (no error)"=w378, "instrument handle"=w375) -> ("error out"=w372:errorcluster, "Measurement"=w368:dbl, "instrument handle out"=w373:refnum<k15>)  [unwired: 7 in]
        "Current, A" <- w368
        n160 = Fract/Exp String To Number(string="NI DMM 1 units 3") -> (number=w376:dbl)  [unwired: 3 in, 1 out]
        n161 = Multiply(x=w376, y=w368) -> (x*y=w369:dbl)
        n162 = Absolute Value(x=w369) -> (abs(x)=→"Current Char":dbl)
        n163 = Absolute Value(x=w369) -> (abs(x)=→"Current":dbl)
        n164 = local read "Стоп"() -> (w374:bool)
      }
    }
    n165 = call <vilib>:"Simple Error Handler.vi"("error in (no error)"=w352) -> ("error out"=w357:errorcluster)  [unwired: 1 in, 7 out]
  }
  n166 = while {
    tunnel: w2 -> [w380]
    tunnel: w5 -> [w382]
    tunnel: [w380] -> w9
    tunnel: w3 -> [w383]
    stop <- w379 stop-if-true
    # "Управление шаговым двигателем"
    n167 = Wait (ms)(milliseconds to wait=u32 1) -> ()  [unwired: 1 out]
    n168 = event shown="[0] \"Погнали!\": Value Change" {
      selector: _ -> [_ _ _]
      dyn-events: _ -> [_ _ _]
      timeout: _ -> [_ _ _]
      tunnel: w380 -> [w388 w416 _]
      tunnel: w383 -> [w387 _ _]
      tunnel: w382 -> [w386 _ _]
      tunnel: [_ _ w422] -> w379
      event "Погнали!": Value Change {
        n169 = event-data() -> ("NewVal"=w384:bool)  [unwired: 1 in, 5 out]
        n170 = case shown="True" w384 {
          tunnel: "Go To" -> [_ w392]
          tunnel: w388 -> [_ w391]
          tunnel: w387 -> [_ _]
          tunnel: w386 -> [_ w390]
          frame False {
            n171 = Wait (ms)(milliseconds to wait=u32 1) -> ()  [unwired: 1 out]
          }
          frame True {
            n172 = while {
              tunnel: w392 -> [w399]
              tunnel: w391 -> [w400]
              tunnel: w390 -> [w402]
              stop <- w403 stop-if-true
              n173 = invoke class="AmateurStepperMotor" method="GoTo"(reference=w400, "destinationPosition"=w399) -> (reference out=w395:refnum<k24>, "GoTo"=w398:refnum<k24>)  [unwired: 2 in, 2 out]
              n174 = invoke class="Task" method="ConfigureAwait"(reference=w398, "continueOnCapturedContext"=FALSE) -> ()  [unwired: 2 in, 4 out]
              n175 = Wait (ms)(milliseconds to wait=u32 1) -> ()  [unwired: 1 out]
              n176 = while {
                tunnel: [w404] -> _
                tunnel: [w406] -> w396
                tunnel: [w408] -> w403
                tunnel: w399 -> [w413]
                tunnel: w402 -> [w411]
                tunnel: w395 -> [w405]
                stop <- w408 stop-if-true
                n177 = property class="AmateurStepperMotor"(reference=w405) -> (reference out=w406:refnum<k24>, "Position"=w404:dbl)  [unwired: 1 in, 1 out]
                "Position" <- w404
                n178 = Subtract(x=w404, y=w413) -> (x-y=w414:dbl)
                n179 = Wait (ms)(milliseconds to wait=u32 1) -> ()  [unwired: 1 out]
                n180 = Absolute Value(x=w414) -> (abs(x)=w412:dbl)
                n181 = Less Or Equal?(x=w412, y=w411) -> (x <= y?=w410:bool)
                n182 = Or(x=w410, y="Стоп GoTo") -> (x .or. y?=w408:bool)
                "Готово" <- w408
              }
              n183 = invoke class="AmateurStepperMotor" method="Stop"(reference=w396) -> (reference out=w394:refnum<k24>)  [unwired: 2 in, 2 out]
              n184 = property class="AmateurStepperMotor"(reference=w394) -> ("Position"=w393:dbl)  [unwired: 1 in, 2 out]
              n185 = local write "Position"(w393) -> ()
            }
          }
        }
      }
      event "set pos": Value Change {
        n186 = event-data() -> ("NewVal"=w417:bool)  [unwired: 1 in, 5 out]
        n187 = case shown="False" w417 {
          tunnel: w416 -> [_ w421]
          tunnel: "new pos" -> [_ w420]
          frame False {
          }
          frame True {
            n188 = property class="AmateurStepperMotor"(reference=w421, "Position"=w420) -> (reference out=w419:refnum<k24>)  [unwired: 1 in, 1 out]
            n189 = property class="AmateurStepperMotor"(reference=w419) -> ("Position"=w418:dbl)  [unwired: 1 in, 2 out]
            n190 = local write "Position"(w418) -> ()
          }
        }
      }
      event "Стоп": Value Change {
        n191 = event-data() -> ()  [unwired: 1 in, 6 out]
        n192 = local read "Стоп"() -> (w422:bool)
      }
    }
  }
  n193 = while {
    shift-right: [w425] -> _
    shift-left: 0 -> [w426]
    tunnel: w41 -> [_]
    stop <- w429 stop-if-true
    # "Управление Ардуино тумблерами"
    n194 = local read "Стоп"() -> (w429:bool)
    n195 = Wait (ms)(milliseconds to wait=u32 10 ("millisecond timer value")) -> ()  [unwired: 1 out]
    n196 = Boolean Array To Number(Boolean array="Сегменты") -> (number=w424:u32)
    n197 = To Long Integer(number=w424) -> (32bit integer=w425:i32)
    n198 = Not Equal?(x=w425, y=w426) -> (x != y?=w427:bool)
    n199 = case shown="True" w427 {
      tunnel: w425 -> [_ w430]
      tunnel: w426 -> [_ w431]
      frame False {
      }
      frame True {
        n200 = stacked-sequence {
          seq-local: [w434 _ _] -> [_ w445 _]
          seq-local: [w432 _ _] -> [_ w440 _]
          seq-local: [_ w441 _] -> [_ _ w481]
          tunnel: w430 -> [w436 _ _]
          tunnel: w431 -> [w435 _ _]
          frame #0 {
            # "Детектирвоание позиции и\nнаправления изменения бита"
            n201 = Subtract(x=w436, y=w435) -> (x-y=w437:i32)
            n202 = To Double Precision Float(number=w437) -> (double precision float=w438:dbl)
            n203 = Greater Than 0?(x=w437) -> (x > 0?=w434:bool)
            "+/-" <- w434
            n204 = Absolute Value(x=w438) -> (abs(x)=w433:dbl)
            n205 = Logarithm Base 2(1:w433) -> (0:w432:dbl)
            "Разряд" <- w432
          }
          frame #1 {
            # "Указывает на последнюю нажатую кнопку"
            # "Выбор бита и направления\n его измнения"
            n206 = case shown="10" w440 {
              tunnel: ["D10" "D9" "D5" "D8" "D11" "D12" "A1" "D4" "A5" "A4" "A3" "A2" "A0" "D13" "D3" "All"] -> w443
              tunnel: ["a" "b" "c" "d" "e" "f" "g" "h" "j" "k" "L" "m" "n" "p" "dp" "All"] -> w439
              frame 0, Default {
                # "a = D10"
              }
              frame 1 {
                # "b = D9"
              }
              frame 2 {
                # "c = D5"
              }
              frame 3 {
                # "d = D8"
              }
              frame 4 {
                # "e = D11"
              }
              frame 5 {
                # "f = D12"
              }
              frame 6 {
                # "g = A1"
              }
              frame 7 {
                # "h = D4"
              }
              frame 8 {
                # "j = A5"
              }
              frame 9 {
                # "k = A4"
              }
              frame 10 {
                # "L = A3"
              }
              frame 11 {
                # "m = A2"
              }
              frame 12 {
                # "n = A0"
              }
              frame 13 {
                # "p = D13"
              }
              frame 14 {
                # "dp = D3"
              }
              frame 15 {
              }
            }
            "Сегмент" <- w439
            n207 = Select(t="off", s=w445, f="on") -> (s? t:f=w442:string)
            n208 = Concatenate Strings(w443, "_" ("string"), w442) -> (w441:string)
          }
          frame #2 {
            # "Передача команды в Ардуино"
            n209 = Equal?(x=w481, y="All_off") -> (x = y?=w484:bool)
            n210 = Equal?(x=w481, y="All_on") -> (x = y?=w482:bool)
            n211 = case shown="True" w484 {
              frame False {
              }
              frame True {
                n212 = local write "Сегменты"(bool[] [TRUE, TRUE, TRUE, TRUE, TRUE, TRUE, TRUE, TRUE, TRUE, TRUE, TRUE, TRUE, TRUE, TRUE, TRUE, TRUE] ("Сегменты")) -> ()
              }
            }
            n213 = case shown="True" w482 {
              frame False {
              }
              frame True {
                n214 = local write "Сегменты"(bool[] [FALSE, FALSE, FALSE, FALSE, FALSE, FALSE, FALSE, FALSE, FALSE, FALSE, FALSE, FALSE, FALSE, FALSE, FALSE, FALSE] ("Сегменты")) -> ()
              }
            }
            n215 = stacked-sequence {
              tunnel: w481 -> [w487 _ _]
              frame #0 {
                n216 = local write "Command"(w487) -> ()
              }
              frame #1 {
                n217 = local write "Записать"(TRUE ("Записать")) -> ()
                n218 = Wait (ms)(milliseconds to wait=u32 1000) -> ()  [unwired: 1 out]
              }
              frame #2 {
                n219 = local write "Записать"(FALSE ("Записать")) -> ()
                n220 = Wait (ms)(milliseconds to wait=u32 1000) -> ()  [unwired: 1 out]
              }
            }
          }
        }
      }
    }
  }
  n221 = call <instrlib>:"niDMM Close.vi"("error in (no error)"=w34, "instrument handle"=w35) -> ()  [unwired: 9 in, 1 out]
  n222 = while {
    tunnel: [w498] -> w36
    tunnel: w39 -> [w496]
    tunnel: w38 -> [w495]
    tunnel: [w492] -> w37
    stop <- w494 stop-if-true
    # "Настройка вольтметра NI PXI-4071"
    n223 = Wait (ms)(milliseconds to wait=u32 1) -> ()  [unwired: 1 out]
    n224 = flat-sequence {
      tunnel: [w505] -> w500
      tunnel: w496 -> [w503]
      tunnel: w495 -> [w507]
      tunnel: [w504] -> w499
      tunnel: w500 -> [w516]
      tunnel: w499 -> [w519]
      tunnel: [w515] -> w494
      tunnel: [w514] -> w492
      tunnel: [w513] -> w493
      frame #0 {
        w501 = T6 6.5 items=["3 1/2"=3.5, "4 1/2"=4.5, "5 1/2"=5.5, "6 1/2"=6.5, "7 1/2"=7.5] ("Resolution in Digits")
        n225 = Fract/Exp String To Number(string="NI DMM 1 Voltage Range 4") -> (number=w506:dbl)  [unwired: 3 in, 1 out]
        n226 = call-poly <instrlib>:"niDMM Config Measurement.vi"("Range"=w506, "Resolution in Digits"=w501, "error in (no error)"=w507, "Function"=niDMM_Function."DC Volts" ("Measurement Type"), "instrument handle"=w503) -> ("error out"=w504:errorcluster, "instrument handle out"=w505:refnum<k15>)  [unwired: 5 in]
      }
      frame #1 {
        n227 = call <instrlib>:"niDMM Read.vi"("error in (no error)"=w519, "instrument handle"=w516) -> ("error out"=w513:errorcluster, "Measurement"=w511:dbl, "instrument handle out"=w514:refnum<k15>)  [unwired: 7 in]
        "Voltage, V" <- w511
        n228 = Fract/Exp String To Number(string="NI DMM 1 units 4") -> (number=w517:dbl)  [unwired: 3 in, 1 out]
        n229 = Multiply(x=w517, y=w511) -> (x*y=w509:dbl)
        n230 = Absolute Value(x=w509) -> (abs(x)=→"Voltage Char":dbl)
        n231 = Absolute Value(x=w509) -> (abs(x)=→"Voltage":dbl)
        n232 = local read "Стоп"() -> (w515:bool)
      }
    }
    n233 = call <vilib>:"Simple Error Handler.vi"("error in (no error)"=w493) -> ("error out"=w498:errorcluster)  [unwired: 1 in, 7 out]
  }
  n234 = invoke class="AmateurStepperMotor" method="Stop"(reference=w9) -> (reference out=w16:refnum<k24>, "Stop"=w17:refnum<k24>)  [unwired: 2 in, 1 out]
  n235 = property class="AmateurStepperMotor"(reference=w16, "HoldOn"=FALSE) -> (reference out=w15:refnum<k24>)  [unwired: 1 in, 1 out]
  n236 = invoke class="AmateurStepperMotor" method="Dispose"(reference=w15) -> (error out=w12:errorcluster)  [unwired: 2 in, 2 out]
  n237 = invoke class="SerialPort" method="Close"(reference=w27, error in=w12) -> (reference out=w11:refnum<k24>, error out=w13:errorcluster)  [unwired: 1 in, 1 out]
  n238 = invoke class="Task" method="Wait"(reference=w17) -> ()  [unwired: 2 in, 3 out]
  n239 = Close Reference(reference=w11, error in (no error)=w13) -> (error out=w14:errorcluster)
  n240 = call <vilib>:"Simple Error Handler.vi"("error in (no error)"=w14) -> ()  [unwired: 1 in, 8 out]
  n241 = VISA Close(VISA resource name=w20, error in (no error)=w19) -> (error out=w29:errorcluster)
  n242 = call <instrlib>:"niDMM Close.vi"("error in (no error)"=w36, "instrument handle"=w37) -> ()  [unwired: 9 in, 1 out]
  n243 = call <instrlib>:"niDCPower Close.vi"("instrument handle"=w42) -> ()  [unwired: 10 in, 1 out]
  n244 = call "Ophir Error Message.vi"("error in (no error)"=w29) -> ()  [unwired: 3 in, 4 out]
